vi "PRL UTIL Calculate Activity.vi"(2 "Data Indicator":i32, 3 "Init?":bool) -> (0 "Activity Monitor":dbl, 1 "Refresh?":bool)   [LabVIEW 2018, in "S3DK.lvlib" / "PMU Recorder Light.lvlib"]
doc: "Keeps a buffer of the data indicator (0 means no data, 1 means data). Then, based on the values present in the buffer, it calculates the percentage of requests to the dll that has resulted in data being recieved. This is an indicator of how well the computer is handelling data processing, and if there is data coming in at all."
uses:
  PMU Recorder Light.lvlib
  Setting Choice.ctl
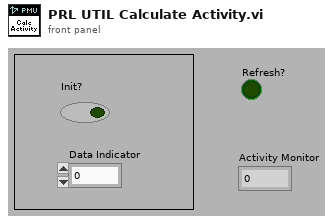
[diagram p1: front panel]
types:
  T1 = typedef "S3DK.lvlib/PMU Recorder Light.lvlib/Setting Choice.ctl" = enum16{"Analog Data Points Allowed Equals", "Complex Data Points Allowed Equals", "Seconds Before Reset After Wait for Config Fails", "Number of Live Buffer in Access Buffer ", "Number of Connection Attempts", "Live Data Buffer Size", "dt Tolerance", "Data Rate History", "ALL"}
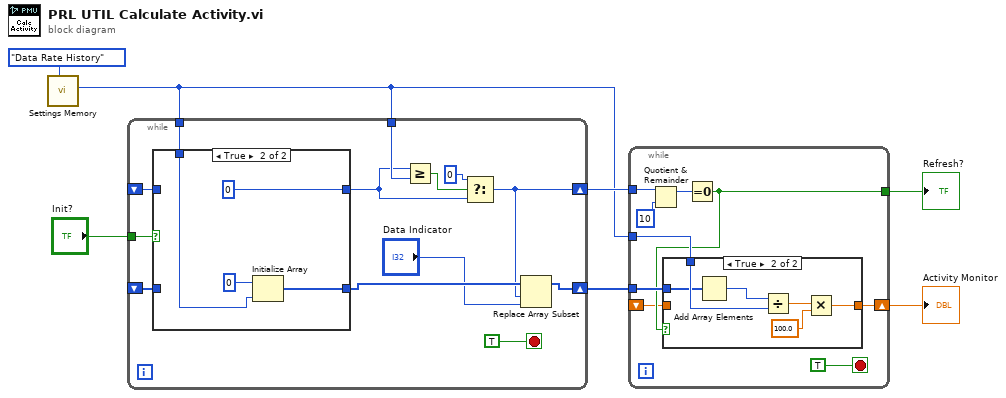
[diagram p0: block diagram]
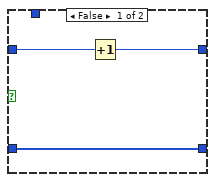
[diagram p3: hidden frame]
diagram:
  n1 = call "Settings Memory.vi"("Setting Choice"=Setting_Choice."Data Rate History") -> ("Output Int32"=w1:i32)  [unwired: 8 in, 2 out]
  n2 = while {
    tunnel: "Init?" -> [w20]
    shift-right: [w10] -> w6
    shift-left: _ -> [w19]
    tunnel: w1 -> [w18]
    shift-right: [w8] -> w5
    shift-left: _ -> [w16]
    tunnel: w1 -> [w15]
    stop <- TRUE stop-if-true
    n3 = case shown="True" w20 {
      tunnel: [w23 w25] -> w11
      tunnel: w19 -> [w23 _]
      tunnel: w18 -> [_ w27]
      tunnel: w16 -> [w22 _]
      tunnel: [w21 0] -> w12
      frame False {
        n4 = Increment(x=w22) -> (x+1=w21:i32)
      }
      frame True {
        n5 = Initialize Array(0, w27) -> (w25:i32[])
      }
    }
    n6 = Greater Or Equal?(x=w12, y=w15) -> (x >= y?=w13:bool)
    n7 = Select(t=0, s=w13, f=w12) -> (s? t:f=w8:i32)
    n8 = Replace Array Subset(array=w11, new element="Data Indicator", index=w8) -> (w10:i32[])
  }
  n9 = while {
    tunnel: w1 -> [w35]
    tunnel: w6 -> [w34]
    tunnel: w5 -> [w32]
    shift-right: [w36] -> w4
    shift-left: _ -> [w29]
    tunnel: [w30] -> w3
    stop <- TRUE stop-if-true
    n10 = Quotient & Remainder(x=w32, y=10) -> (x-y*floor(x/y)=w31:i32)  [unwired: 1 out]
    n11 = Equal To 0?(x=w31) -> (x = 0?=w30:bool)
    n12 = case shown="True" w30 {
      tunnel: [w37 w40] -> w36
      tunnel: w35 -> [_ w39]
      tunnel: w34 -> [_ w38]
      tunnel: w29 -> [w37 _]
      frame False {
      }
      frame True {
        n13 = Add Array Elements(numeric array=w38) -> (sum=w43:i32)
        n14 = Divide(x=w43, y=w39) -> (x/y=w42:dbl)
        n15 = Multiply(x=w42, y=100.0) -> (x*y=w40:dbl)
      }
    }
  }
  "Activity Monitor" <- w4
  "Refresh?" <- w3
